vi "svx_Timebase Update Pair.vi"(6 "State in":T1={"X Scale"={"Name"="Time", "FString"="%#.2g", "Major Color"=16777238, "Minor Color"=16777216, "Grid Style"=1, "Maximum"=0.5, "Minimum"=0.0, "Autoscale"=TRUE, "Show Scale Label"={"Probe X"=FALSE, "Probe Y"=TRUE}, "Show Scale"={"Probe X"=TRUE, "Probe Y"=TRUE}, "Autoscale Once"=FALSE}, "Y Scale"={"Name"="Amplitude", "FString"="%#.2g", "Major Color"=16777238, "Minor Color"=16777216, "Scale Visible"=TRUE, " Label Visible"=TRUE, "Grid Style"=1, "Autoscale"=TRUE, "Maximum"={"Probe X"=1.0, "Probe Y"=1.0}, "Minimum"={"Probe X"=-1.0, "Probe Y"=-1.0}, "Autoscale Once"=FALSE}, "Plot"={"Point Style"=0, "Line Width"=0, "Line Style"=0, "Plot Color"=16860, "Point/fill"=16860}, "Tacho Point Color"=16711680, "Property Name"=[], "Container Bounds"={"Width"=640, "Height"=360}, "Background color"=16777226, "Legend Visible"=TRUE, "Scale Range Change"=refnum, "Strings[]"={"Custom pair name"=FALSE, "Row Strings []"=[], "Column Strings []"=[]}, "Cursor"={"Cursor Point Style"=13, "Cursor Style"=5, "Cursor Line Width"=1, "Cursor Line Style"=0, "Cursor Color"=16860, "Cursor Name Visible"=TRUE, "Cursor Visible"=TRUE, "Cursor Lock"=FALSE, "Cursor Index"=0}, "Index"=[], "Legend Width"=200, " Parents Tags"=[], "Children Tags"=[], "Open?"=[], "Label"="Timebase Plot", "Cursor X Pos"={"X"=0.0, "Y"=0.0}, "Cursor Y Pos"={"X"=0.0, "Y"=0.0}, "Graph Type"=enum."Probe X and Y", "Prev Graph Type"=enum."Probe X and Y", "Prev Legend Visible"=TRUE, "Cursor Release"=refnum, "Pair Strings Changed?"=FALSE, "Cursor ID"=refnum, "Legend Background"=16777226, "Legend Font"=16777222, "Probe Y Label"="Probe Y", "Probe X Label"="Probe X", "Probe X Label Visible"=TRUE, "Probe Y Label Visible"=TRUE, "Tree Item Width"=200, "# Custom RowStr"=0, "# Custom ColStr"=0, "Property Name"=refnum, "Data Related State"=refnum} caption="State", 10 "Label Text":string, 11 "timebase plot":T5) -> (0 "update tree?":bool, 4 "State out":T1={"X Scale"={"Name"="Time", "FString"="%#.2g", "Major Color"=16777238, "Minor Color"=16777216, "Grid Style"=1, "Maximum"=0.5, "Minimum"=0.0, "Autoscale"=TRUE, "Show Scale Label"={"Probe X"=FALSE, "Probe Y"=TRUE}, "Show Scale"={"Probe X"=TRUE, "Probe Y"=TRUE}, "Autoscale Once"=FALSE}, "Y Scale"={"Name"="Amplitude", "FString"="%#.2g", "Major Color"=16777238, "Minor Color"=16777216, "Scale Visible"=TRUE, " Label Visible"=TRUE, "Grid Style"=1, "Autoscale"=TRUE, "Maximum"={"Probe X"=1.0, "Probe Y"=1.0}, "Minimum"={"Probe X"=-1.0, "Probe Y"=-1.0}, "Autoscale Once"=FALSE}, "Plot"={"Point Style"=0, "Line Width"=0, "Line Style"=0, "Plot Color"=16860, "Point/fill"=16860}, "Tacho Point Color"=16711680, "Property Name"=[], "Container Bounds"={"Width"=640, "Height"=360}, "Background color"=16777226, "Legend Visible"=TRUE, "Scale Range Change"=refnum, "Strings[]"={"Custom pair name"=FALSE, "Row Strings []"=[], "Column Strings []"=[]}, "Cursor"={"Cursor Point Style"=13, "Cursor Style"=5, "Cursor Line Width"=1, "Cursor Line Style"=0, "Cursor Color"=16860, "Cursor Name Visible"=TRUE, "Cursor Visible"=TRUE, "Cursor Lock"=FALSE, "Cursor Index"=0}, "Index"=[], "Legend Width"=200, " Parents Tags"=[], "Children Tags"=[], "Open?"=[], "Label"="Timebase Plot", "Cursor X Pos"={"X"=0.0, "Y"=0.0}, "Cursor Y Pos"={"X"=0.0, "Y"=0.0}, "Graph Type"=enum."Probe X and Y", "Prev Graph Type"=enum."Probe X and Y", "Prev Legend Visible"=TRUE, "Cursor Release"=refnum, "Pair Strings Changed?"=FALSE, "Cursor ID"=refnum, "Legend Background"=16777226, "Legend Font"=16777222, "Probe Y Label"="Probe Y", "Probe X Label"="Probe X", "Probe X Label Visible"=TRUE, "Probe Y Label Visible"=TRUE, "Tree Item Width"=200, "# Custom RowStr"=0, "# Custom ColStr"=0, "Property Name"=refnum, "Data Related State"=refnum} caption="State")   [LabVIEW 2017, in "SVX Timebase.xctl"]
uses:
  <vilib>/addons/_XControls/Timebase Plot/SVX Timebase.xctl
  <vilib>/addons/_XControls/Timebase Plot/subVIs/svx_Timebase Data.ctl
  <vilib>/addons/_XControls/Timebase Plot/subVIs/svx_Timebase State.ctl
  <vilib>/addons/_XControls/Timebase Plot/subVIs/svx_Timebase Bounds.ctl
  <vilib>/addons/_XControls/Timebase Plot/subVIs/svx_Timebase Graph Types.ctl
  <vilib>/addons/_XControls/Timebase Plot/subVIs/svx_Timebase Data Related State.ctl
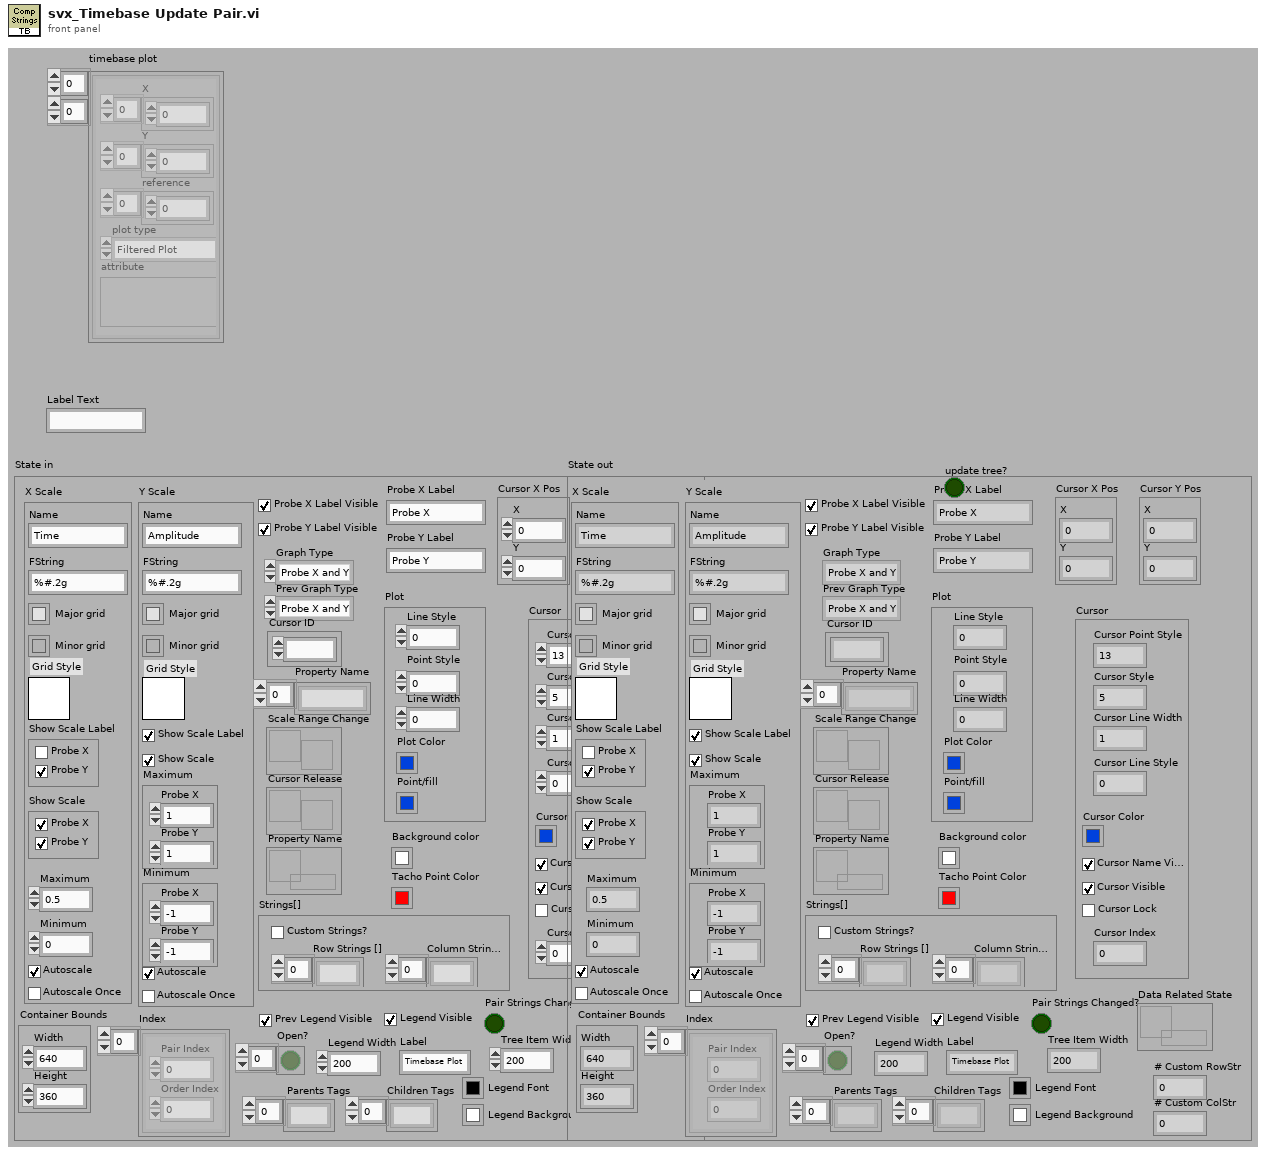
[diagram p1: front panel]
types:
  T1 = typedef "SVX Timebase.xctl/svx_Timebase State.ctl" = cluster{"X Scale":cluster{"Name":string, "FString":string, "Major Color":u32, "Minor Color":u32, "Grid Style":u16, "Maximum":dbl, "Minimum":dbl, "Autoscale":bool, "Show Scale Label":cluster{"Probe X":bool, "Probe Y":bool}, "Show Scale":cluster{"Probe X":bool, "Probe Y":bool}, "Autoscale Once":bool}, "Y Scale":cluster{"Name":string, "FString":string, "Major Color":u32, "Minor Color":u32, "Scale Visible":bool, " Label Visible":bool, "Grid Style":u16, "Autoscale":bool, "Maximum":cluster{"Probe X":dbl, "Probe Y":dbl}, "Minimum":cluster{"Probe X":dbl, "Probe Y":dbl}, "Autoscale Once":bool}, "Plot":cluster{"Point Style":u8, "Line Width":u8, "Line Style":u8, "Plot Color":u32, "Point/fill":u32}, "Tacho Point Color":u32, "Property Name":string[], "Container Bounds":T2, "Background color":u32, "Legend Visible":bool, "Scale Range Change":refnum<user-event>, "Strings[]":cluster{"Custom pair name":bool, "Row Strings []":string[], "Column Strings []":string[]}, "Cursor":cluster{"Cursor Point Style":u8, "Cursor Style":u8, "Cursor Line Width":u8, "Cursor Line Style":u8, "Cursor Color":u32, "Cursor Name Visible":bool, "Cursor Visible":bool, "Cursor Lock":bool, "Cursor Index":i32}, "Index":cluster{"Pair Index":u32, "Order Index":u32}[], "Legend Width":u32, " Parents Tags":string[], "Children Tags":string[], "Open?":bool[], "Label":string, "Cursor X Pos":cluster{"X":dbl, "Y":dbl}, "Cursor Y Pos":cluster{"X":dbl, "Y":dbl}, "Graph Type":T3, "Prev Graph Type":T3, "Prev Legend Visible":bool, "Cursor Release":refnum<user-event>, "Pair Strings Changed?":bool, "Cursor ID":refnum<k1>, "Legend Background":u32, "Legend Font":u32, "Probe Y Label":string, "Probe X Label":string, "Probe X Label Visible":bool, "Probe Y Label Visible":bool, "Tree Item Width":u32, "# Custom RowStr":u32, "# Custom ColStr":u32, "Property Name":refnum<queue>, "Data Related State":T4}
  T2 = typedef "SVX Timebase.xctl/svx_Timebase Bounds.ctl" = cluster{"Width":u32, "Height":u32}
  T3 = typedef "SVX Timebase.xctl/svx_Timebase Graph Types.ctl" = enum16{"Probe X", "Probe Y", "Probe X and Y"}
  T4 = typedef "SVX Timebase.xctl/svx_Timebase Data Related State.ctl" = refnum<queue>
  T5 = typedef "SVX Timebase.xctl/svx_Timebase Data.ctl" = cluster{"X":dbl[], "Y":dbl[], "reference":dbl[], "plot type":enum16{"Filtered Plot", "Unfiltered Plot"}, "attribute":variant}[][]
  T6 = cluster{"X":dbl[], "Y":dbl[], "reference":dbl[], "plot type":enum16{"Filtered Plot", "Unfiltered Plot"}, "attribute":variant}
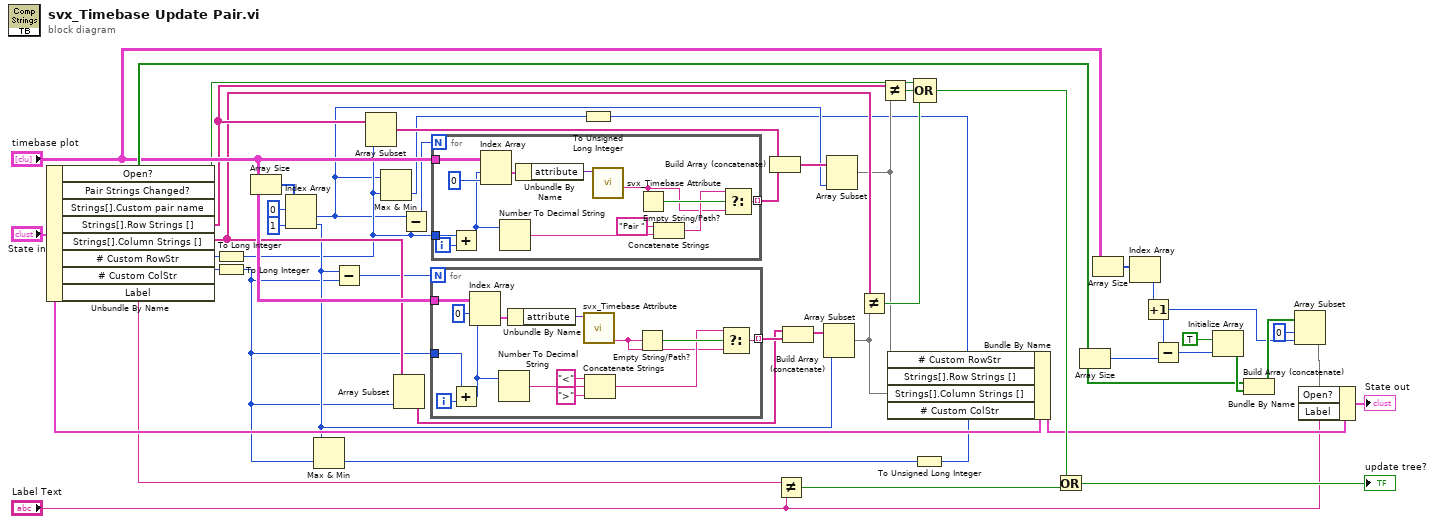
[diagram p0: block diagram]
diagram:
  n1 = Unbundle By Name("State in") -> ("Open?"=w35:bool[], "Pair Strings Changed?"=w1:bool, "Strings[].Row Strings []"=w24:string[], "Strings[].Column Strings []"=w23:string[], "# Custom RowStr"=w20:u32, "# Custom ColStr"=w15:u32, "Label"=w47:string)  [unwired: 1 out]
  n2 = To Long Integer(number=w20) -> (32bit integer=w6:i32)
  n3 = To Long Integer(number=w15) -> (32bit integer=w9:i32)
  n4 = Array Size(array="timebase plot") -> (size(s)=w29:i32[])
  n5 = Index Array(array=w29, index #1=0 ("index"), index #2=1 ("index")) -> (element #1=w5:i32, element #2=w10:i32)
  n6 = Max & Min(x=w10, y=w9) -> (min(x,y)=w8:i32)  [unwired: 1 out]
  n7 = Subtract(x=w10, y=w9) -> (x-y=w19:i32)
  n8 = Array Subset(array=w24, length=w6) -> (w17:string[])  [unwired: 1 in]
  n9 = Max & Min(x=w5, y=w6) -> (min(x,y)=w4:i32)  [unwired: 1 out]
  n10 = Array Subset(array=w23, length=w9) -> (w16:string[])  [unwired: 1 in]
  n11 = Subtract(x=w5, y=w6) -> (x-y=w18:i32)
  n12 = for {
    N: w19 -> [_]
    tunnel: "timebase plot" -> [w62]
    tunnel: [w55] -> w25 mode=indexing
    tunnel: w9 -> [w53]
    i -> [w61]
    n13 = Add(x=w53, y=w61) -> (x+y=w54:i32)
    n14 = Index Array(array=w62, index (row)=0 ("disabled index (row)"), index (col)=w54) -> (element=w59:T6)
    n15 = Number To Decimal String(number=w54) -> (decimal integer string=w56:string)  [unwired: 1 in]
    n16 = Unbundle By Name(w59) -> ("attribute"=w52:variant)
    n17 = call <vilib>:"svx_Timebase Attribute.vi"("attribute"=w52) -> ("order"=w49:string)  [unwired: 8 in, 2 out]
    n18 = Concatenate Strings("<" ("string"), w56, ">" ("string")) -> (w50:string)
    n19 = Empty String/Path?(string/path=w49) -> (empty?=w51:bool)
    n20 = Select(t=w50, s=w51, f=w49) -> (s? t:f=w55:string)
  }
  n21 = for {
    N: w18 -> [_]
    tunnel: "timebase plot" -> [w74]
    tunnel: [w67] -> w26 mode=indexing
    tunnel: w6 -> [w69]
    i -> [w70]
    n22 = Add(x=w69, y=w70) -> (x+y=w71:i32)
    n23 = Index Array(array=w74, index (row)=w71, index (col)=0 ("disabled index (col)")) -> (element=w73:T6)
    n24 = Number To Decimal String(number=w71) -> (decimal integer string=w68:string)  [unwired: 1 in]
    n25 = Unbundle By Name(w73) -> ("attribute"=w65:variant)
    n26 = call <vilib>:"svx_Timebase Attribute.vi"("attribute"=w65) -> ("pair"=w63:string)  [unwired: 8 in, 2 out]
    n27 = Empty String/Path?(string/path=w63) -> (empty?=w66:bool)
    n28 = Concatenate Strings("Pair " ("string"), w68) -> (w64:string)
    n29 = Select(t=w64, s=w66, f=w63) -> (s? t:f=w67:string)
  }
  n30 = To Unsigned Long Integer(number=w4) -> (unsigned 32bit integer=w3:u32)
  n31 = Build Array (concatenate)(w17, w26) -> (w14:string[])
  n32 = Not Equal?(x=w47, y="Label Text") -> (x != y?=w2:bool)
  n33 = Build Array (concatenate)(w16, w25) -> (w12:string[])
  n34 = Array Subset(array=w12, length=w10) -> (w11:string[])  [unwired: 1 in]
  n35 = Array Subset(array=w14, length=w5) -> (w13:string[])  [unwired: 1 in]
  n36 = Not Equal?(x=w23, y=w11) -> (x != y?=w27:bool)
  n37 = Not Equal?(x=w24, y=w13) -> (x != y?=w28:bool)
  n38 = Compound Arithmetic op=OR(w1, w28, w27) -> (w46:bool)
  n39 = To Unsigned Long Integer(number=w8) -> (unsigned 32bit integer=w7:u32)
  n40 = Bundle By Name(cluster="State in", "# Custom RowStr"=w3, "Strings[].Row Strings []"=w13, "Strings[].Column Strings []"=w11, "# Custom ColStr"=w7) -> (w44:T1)
  n41 = Or(x=w46, y=w2) -> (x .or. y?=→"update tree?":bool)
  n42 = Array Size(array=w35) -> (size(s)=w41:i32)
  n43 = Array Size(array="timebase plot") -> (size(s)=w33:i32[])
  n44 = Index Array(array=w33) -> (element=w31:i32)  [unwired: 1 in]
  n45 = Increment(x=w31) -> (x+1=w30:i32)
  n46 = Subtract(x=w30, y=w41) -> (x-y=w40:i32)
  n47 = Initialize Array(TRUE ("x .or. y?"), w40) -> (w38:bool[])
  n48 = Build Array (concatenate)(w35, w38) -> (w37:bool[])
  n49 = Array Subset(array=w37, index=0, length=w30) -> (w32:bool[])
  n50 = Bundle By Name(cluster=w44, "Open?"=w32, "Label"="Label Text") -> (→"State out":T1)
